vi "3D-InitialParam.vi"(0 "名称或相对路径":string) -> (3 "Motion Param Cal  Title":string[](array[string]), 4 "Version Param Out":string[][](array[string]) caption="Vision Params", 6 "Motion Param Out":string[][](array[string]) caption="Motion Params", 10 "Modbus Param Out":string[][](array[string]), 14 "Motion Param Cal Out":string[][](array[string]), 15 "List Param Out":string[][](array[string]))   [LabVIEW 2017]
uses:
  Global System.vi
  <vilib>/Utility/file.llb/Read From Spreadsheet File (string).vi
panel:
  out "添加的路径":path
  # "D:\\KNight Back Housing\\Source Code\\Template Program\\potteryTemplete"
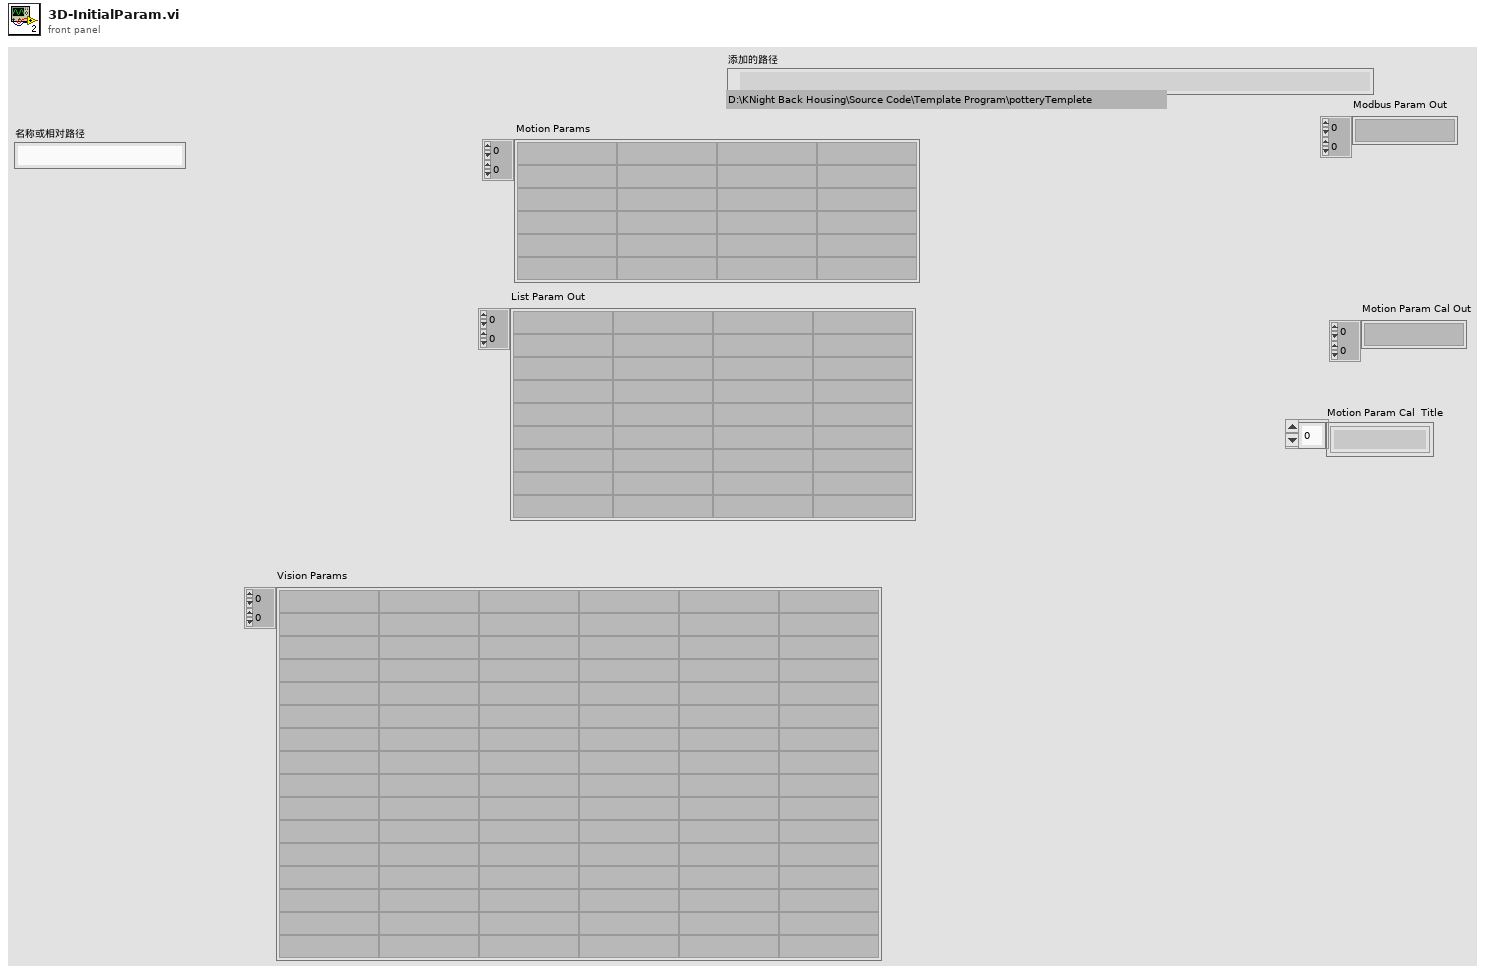
[diagram p1: front panel]
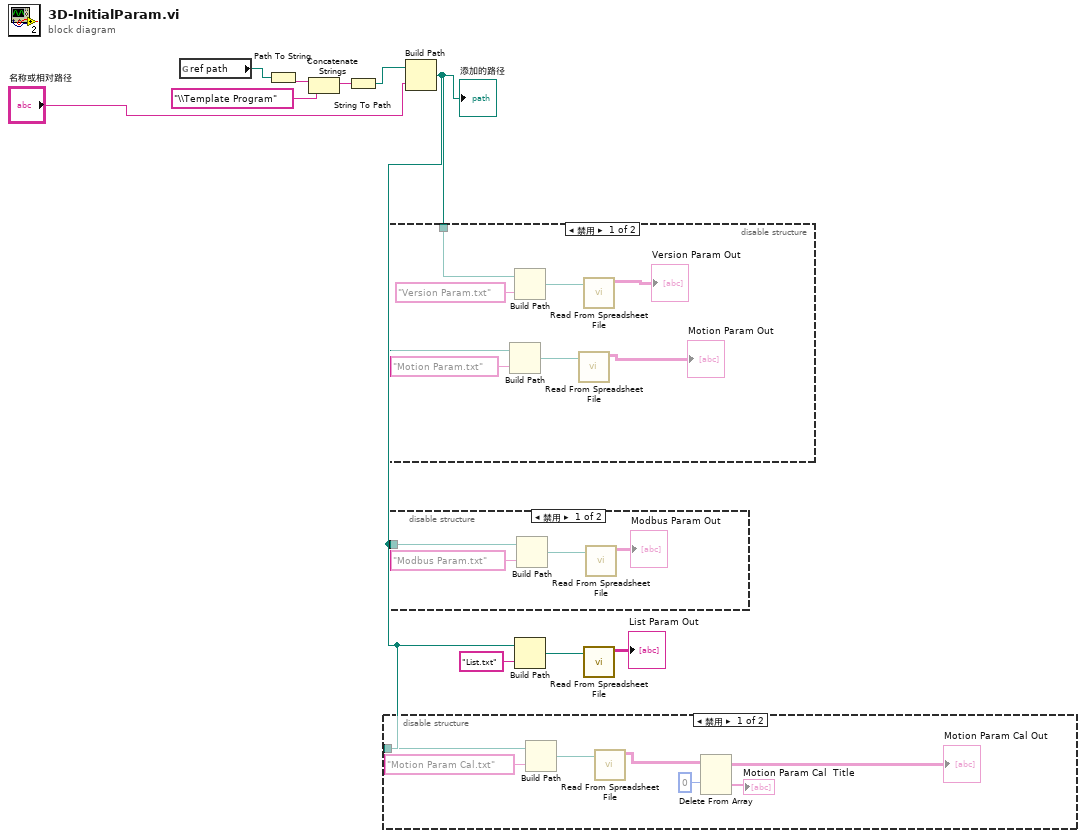
[diagram p0: block diagram]
diagram:
  n1 = global read "Global System.vi" "ref path"() -> (w7:path)
  n2 = Path To String(path=w7) -> (string=w10:string)
  n3 = Concatenate Strings(w10, "\\Template Program" ("字符串")) -> (w8:string)
  n4 = String To Path(string=w8) -> (path=w6:path)
  n5 = Build Path(base path=w6, name or relative path="名称或相对路径") -> (appended path=w1:path)
  "添加的路径" <- w1
  n6 = disable-structure shown="禁用" {
    disable-tunnel: w1 -> [w15 _]
    frame Disabled {
      n7 = Build Path(base path=w15, name or relative path="Motion Param Cal.txt" ("名称或相对路径")) -> (appended path=w16:path)
      n8 = call-poly <vilib>:"Read From Spreadsheet File.vi"("file path (dialog if empty)"=w16) -> ("all rows"=w14:string[][])  [unwired: 6 in, 4 out]
      n9 = Delete From Array(array=w14, index (row)=0 ("索引 (行)")) -> (deleted portion=→"Motion Param Cal  Title":string[], array with subset deleted=→"Motion Param Cal Out":string[][])  [unwired: 2 in]
    }
    frame Enabled {
    }
  }
  n10 = disable-structure shown="禁用" {
    disable-tunnel: w1 -> [w18 _]
    frame Disabled {
      n11 = Build Path(base path=w18, name or relative path="Motion Param.txt" ("名称或相对路径")) -> (appended path=w20:path)
      n12 = Build Path(base path=w18, name or relative path="Version Param.txt" ("名称或相对路径")) -> (appended path=w23:path)
      n13 = call-poly <vilib>:"Read From Spreadsheet File.vi"("file path (dialog if empty)"=w20) -> ("all rows"=→"Motion Param Out":string[][])  [unwired: 6 in, 4 out]
      n14 = call-poly <vilib>:"Read From Spreadsheet File.vi"("file path (dialog if empty)"=w23) -> ("all rows"=→"Version Param Out":string[][])  [unwired: 6 in, 4 out]
    }
    frame Enabled {
    }
  }
  n15 = disable-structure shown="禁用" {
    disable-tunnel: w1 -> [w25 _]
    frame Disabled {
      n16 = Build Path(base path=w25, name or relative path="Modbus Param.txt" ("名称或相对路径")) -> (appended path=w28:path)
      n17 = call-poly <vilib>:"Read From Spreadsheet File.vi"("file path (dialog if empty)"=w28) -> ("all rows"=→"Modbus Param Out":string[][])  [unwired: 6 in, 4 out]
    }
    frame Enabled {
    }
  }
  n18 = Build Path(base path=w1, name or relative path="List.txt" ("名称或相对路径")) -> (appended path=w2:path)
  n19 = call-poly <vilib>:"Read From Spreadsheet File.vi"("file path (dialog if empty)"=w2) -> ("all rows"=→"List Param Out":string[][])  [unwired: 6 in, 4 out]
